vi "诊断标定3.vi"(8 "CAN端口":u16(ring), 9 "设备索引号":u16(ring), 10 "CAN卡类型":u32(ring)=21) -> ()   [LabVIEW 2013] (continued)
                                }
                                }
                                frame 8 {
                                n3916 = case shown="假" w5467 {
                                frame False {
                                n3917 = control-ref of="结果"() -> (w5470:refnum<vi>)
                                n3918 = Build Array("加热控制参数判定失败!") -> (w5471:string[])
                                n3919 = call "表格编辑.vi"("新元素/子数组"=w5471, "活动单元格:单元格背景色"=u32 16711680, "MCListbox引用句柄"=w5470) -> ()  [unwired: 9 out]
                                }
                                frame True {
                                }
                                }
                                }
                                frame 99, Default {
                                }
                                }
                                }
                              }
                            }
                          }
                        }
                        n3920 = disable-structure shown="禁用" {
                          frame Disabled {
                            n3921 = global read "读配置文件全局.vi" "SOC判定"() -> ()  [unwired: 1 out]
                          }
                          frame Enabled {
                          }
                        }
                      }
                    }
                  }
                  frame True {
                  }
                }
              }
            }
            n3922 = stacked-sequence {
              tunnel: w4698 -> [_]
              frame #0 {
                n3923 = local write "强制终止读写标记"(FALSE ("强制停止")) -> ()
              }
            }
            "重试次数" <- u8 0 ("重试次数")
          }
          frame "开启均衡" {
            n3924 = local read "从板板号"() -> (w5472:u8)
            n3925 = stacked-sequence {
              tunnel: 133 -> [_ w5498 _ _]
              tunnel: w5472 -> [_ _ _ _]
              frame #0 {
                w5482 = u8 0 items=["Normal", "Listen Only"] ("工作方式")
                w5481 = u8 1 items=["Dual Filter", "Single Filter"] ("滤波方式")
                n3926 = global write "EV05全局变量1.vi" "读取超时"(FALSE ("读取超时")) -> ()
                n3927 = global write "EV05全局变量1.vi" "流控帧 2"(TRUE ("流控帧 2")) -> ()
                n3928 = local write "写?"(TRUE ("写?")) -> ()
                n3929 = local read "设备索引号"() -> (w5477:u16)
                n3930 = local read "CAN卡类型"() -> (w5476:u32)
                n3931 = local read "CAN端口"() -> (w5478:u16)
                n3932 = local write "控制1"(TRUE ("控制1")) -> ()
                n3933 = local write "消除"(TRUE ("消除")) -> ()
                n3934 = global write "EV05全局变量1.vi" "流控帧"(FALSE ("流控帧")) -> ()
                n3935 = call "CAN_Init-8.6.vi"("CAN卡类型"=w5476, "设备索引号"=w5477, "CAN端口"=w5478, "操作类型"=enum16{"初始化CAN", "关闭CAN"}."初始化CAN", "滤波方式"=w5481, "Accept Code"=u32 606601216, "簇"=T21 {"打开CAN"=FALSE, "初始化CAN"=TRUE, "开始CAN"=TRUE, "重启"=FALSE, "关闭CAN"=FALSE}, "Mask Code"=u32 524287 ("Accept Code"), "工作方式"=w5482, "是否滤波"=TRUE, "滤波选择"=T20 {"fiter_mode"=1, "fiter_endid"=75825152, "fiter_startid"=75890687}) -> ()  [unwired: 3 in, 6 out]
                n3936 = Wait Until Next ms Multiple(millisecond multiple=u32 20 ("毫秒倍数")) -> ()  [unwired: 1 out]
              }
              frame #1 {
                n3937 = local write "命令"(w5498) -> ()
                n3938 = call "ID组合.vi"("SA(4)"=0 ("PDU(1)"), "PS(3)"=63 ("PDU(1)"), "PF(2)"=w5498, "PDU(1)"=4) -> ("ID"=w5497:i32)  [unwired: 7 out]
                n3939 = local read "均衡类型选择"() -> (w5494:enum16{"放电均衡", "充电均衡", "充放电均衡"})
                n3940 = local read "设备索引号"() -> (w5503:u16)
                n3941 = local read "CAN卡类型"() -> (w5504:u32)
                n3942 = local read "CAN端口"() -> (w5502:u16)
                n3943 = local write "命令序号"(2) -> ()
                n3944 = Add(x=w5494, y=1) -> (x+y=w5492:i32)
                n3945 = Build Array(2, 2, w5492) -> (w5505:i32[])
                n3946 = call "transmit-8.6.vi"("can卡类型"=w5504, "设备索引号"=w5503, "CAN端口"=w5502, "ID"=w5497, "SendType"=u8 0, "Data"=w5505) -> ()  [unwired: 3 in, 11 out]
              }
              frame #2 {
                n3947 = Wait Until Next ms Multiple(millisecond multiple=u32 1000 ("毫秒倍数")) -> ()  [unwired: 1 out]
              }
              frame #3 {
                w5513 = u8 0 items=["Normal", "Listen Only"] ("工作方式")
                w5514 = u8 1 items=["Dual Filter", "Single Filter"] ("滤波方式")
                n3948 = global write "EV05全局变量1.vi" "流控帧 2"(FALSE ("流控帧 2")) -> ()
                n3949 = local read "CAN卡类型"() -> (w5519:u32)
                n3950 = local read "设备索引号"() -> (w5518:u16)
                n3951 = local read "CAN端口"() -> (w5517:u16)
                n3952 = local write "控制1"(FALSE ("控制1")) -> ()
                n3953 = local write "消除"(FALSE ("消除")) -> ()
                n3954 = call <vilib>:"Unset Busy.vi"() -> ()  [unwired: 2 in, 10 out]
                n3955 = call "CAN_Init-8.6.vi"("CAN卡类型"=w5519, "设备索引号"=w5518, "CAN端口"=w5517, "操作类型"=enum16{"初始化CAN", "关闭CAN"}."初始化CAN", "滤波方式"=w5514, "Accept Code"=u32 3221225472, "簇"=T21 {"打开CAN"=FALSE, "初始化CAN"=TRUE, "开始CAN"=TRUE, "重启"=FALSE, "关闭CAN"=FALSE}, "Mask Code"=u32 1073741823 ("Accept Code"), "工作方式"=w5513, "是否滤波"=TRUE, "滤波选择"=T20 {"fiter_mode"=1, "fiter_endid"=402653184, "fiter_startid"=419430399}) -> ()  [unwired: 3 in, 6 out]
              }
            }
          }
          frame "关闭均衡" {
            n3956 = local read "从板板号"() -> (w5523:u8)
            n3957 = stacked-sequence {
              tunnel: 133 -> [_ w5547 _ _]
              tunnel: w5523 -> [_ _ _ _]
              frame #0 {
                w5533 = u8 0 items=["Normal", "Listen Only"] ("工作方式")
                w5532 = u8 1 items=["Dual Filter", "Single Filter"] ("滤波方式")
                n3958 = global write "EV05全局变量1.vi" "读取超时"(FALSE ("读取超时")) -> ()
                n3959 = global write "EV05全局变量1.vi" "流控帧 2"(TRUE ("流控帧 2")) -> ()
                n3960 = local write "写?"(TRUE ("写?")) -> ()
                n3961 = local read "设备索引号"() -> (w5528:u16)
                n3962 = local read "CAN卡类型"() -> (w5527:u32)
                n3963 = local read "CAN端口"() -> (w5529:u16)
                n3964 = local write "控制1"(TRUE ("控制1")) -> ()
                n3965 = global write "EV05全局变量1.vi" "流控帧"(FALSE ("流控帧")) -> ()
                n3966 = local write "消除"(TRUE ("消除")) -> ()
                n3967 = call "CAN_Init-8.6.vi"("CAN卡类型"=w5527, "设备索引号"=w5528, "CAN端口"=w5529, "操作类型"=enum16{"初始化CAN", "关闭CAN"}."初始化CAN", "滤波方式"=w5532, "Accept Code"=u32 606601216, "簇"=T21 {"打开CAN"=FALSE, "初始化CAN"=TRUE, "开始CAN"=TRUE, "重启"=FALSE, "关闭CAN"=FALSE}, "Mask Code"=u32 524287 ("Accept Code"), "工作方式"=w5533, "是否滤波"=TRUE, "滤波选择"=T20 {"fiter_mode"=1, "fiter_endid"=75825152, "fiter_startid"=75890687}) -> ()  [unwired: 3 in, 6 out]
                n3968 = Wait Until Next ms Multiple(millisecond multiple=u32 20 ("毫秒倍数")) -> ()  [unwired: 1 out]
              }
              frame #1 {
                n3969 = local write "命令"(w5547) -> ()
                n3970 = call "ID组合.vi"("SA(4)"=0 ("PDU(1)"), "PS(3)"=63 ("PDU(1)"), "PF(2)"=w5547, "PDU(1)"=4) -> ("ID"=w5546:i32)  [unwired: 7 out]
                n3971 = local read "均衡类型选择"() -> (w5557:enum16{"放电均衡", "充电均衡", "充放电均衡"})
                n3972 = local write "命令序号"(3) -> ()
                n3973 = local read "设备索引号"() -> (w5552:u16)
                n3974 = local read "CAN卡类型"() -> (w5553:u32)
                n3975 = local read "CAN端口"() -> (w5551:u16)
                n3976 = Add(x=w5557, y=1) -> (x+y=w5555:i32)
                n3977 = Build Array(2, 3, w5555) -> (w5554:i32[])
                n3978 = call "transmit-8.6.vi"("can卡类型"=w5553, "设备索引号"=w5552, "CAN端口"=w5551, "ID"=w5546, "SendType"=u8 0, "Data"=w5554) -> ()  [unwired: 3 in, 11 out]
              }
              frame #2 {
                n3979 = Wait Until Next ms Multiple(millisecond multiple=u32 1000 ("毫秒倍数")) -> ()  [unwired: 1 out]
              }
              frame #3 {
                w5564 = u8 0 items=["Normal", "Listen Only"] ("工作方式")
                w5565 = u8 1 items=["Dual Filter", "Single Filter"] ("滤波方式")
                n3980 = local read "设备索引号"() -> (w5569:u16)
                n3981 = local read "CAN卡类型"() -> (w5570:u32)
                n3982 = global write "EV05全局变量1.vi" "流控帧 2"(FALSE ("流控帧 2")) -> ()
                n3983 = local read "CAN端口"() -> (w5568:u16)
                n3984 = local write "控制1"(FALSE ("控制1")) -> ()
                n3985 = local write "消除"(FALSE ("消除")) -> ()
                n3986 = call "CAN_Init-8.6.vi"("CAN卡类型"=w5570, "设备索引号"=w5569, "CAN端口"=w5568, "操作类型"=enum16{"初始化CAN", "关闭CAN"}."初始化CAN", "滤波方式"=w5565, "Accept Code"=u32 3221225472, "簇"=T21 {"打开CAN"=FALSE, "初始化CAN"=TRUE, "开始CAN"=TRUE, "重启"=FALSE, "关闭CAN"=FALSE}, "Mask Code"=u32 1073741823 ("Accept Code"), "工作方式"=w5564, "是否滤波"=TRUE, "滤波选择"=T20 {"fiter_mode"=1, "fiter_endid"=402653184, "fiter_startid"=419430399}) -> ()  [unwired: 3 in, 6 out]
                n3987 = call <vilib>:"Unset Busy.vi"() -> ()  [unwired: 2 in, 10 out]
              }
            }
          }
          frame "强制均衡" {
            n3988 = local read "从板板号"() -> (w5574:u8)
            n3989 = stacked-sequence {
              tunnel: 133 -> [_ w5605 _ _]
              tunnel: w5574 -> [_ _ _ _]
              frame #0 {
                w5584 = u8 0 items=["Normal", "Listen Only"] ("工作方式")
                w5583 = u8 1 items=["Dual Filter", "Single Filter"] ("滤波方式")
                n3990 = global write "EV05全局变量1.vi" "读取超时"(FALSE ("读取超时")) -> ()
                n3991 = global write "EV05全局变量1.vi" "流控帧 2"(TRUE ("流控帧 2")) -> ()
                n3992 = local write "写?"(TRUE ("写?")) -> ()
                n3993 = local read "设备索引号"() -> (w5579:u16)
                n3994 = local read "CAN卡类型"() -> (w5578:u32)
                n3995 = local write "控制1"(TRUE ("控制1")) -> ()
                n3996 = local read "CAN端口"() -> (w5580:u16)
                n3997 = local write "消除"(TRUE ("消除")) -> ()
                n3998 = global write "EV05全局变量1.vi" "流控帧"(FALSE ("流控帧")) -> ()
                n3999 = call "CAN_Init-8.6.vi"("CAN卡类型"=w5578, "设备索引号"=w5579, "CAN端口"=w5580, "操作类型"=enum16{"初始化CAN", "关闭CAN"}."初始化CAN", "滤波方式"=w5583, "Accept Code"=u32 606601216, "簇"=T21 {"打开CAN"=FALSE, "初始化CAN"=TRUE, "开始CAN"=TRUE, "重启"=FALSE, "关闭CAN"=FALSE}, "Mask Code"=u32 524287 ("Accept Code"), "工作方式"=w5584, "是否滤波"=TRUE, "滤波选择"=T20 {"fiter_mode"=1, "fiter_endid"=75825152, "fiter_startid"=75890687}) -> ()  [unwired: 3 in, 6 out]
                n4000 = Wait Until Next ms Multiple(millisecond multiple=u32 20 ("毫秒倍数")) -> ()  [unwired: 1 out]
              }
              frame #1 {
                n4001 = local read "强制类型"() -> (w5611:enum16{"全通道开启", "单通道开启", "清待均衡时间"})
                n4002 = case shown="\"清待均衡时间\"" w5611 {
                  tunnel: [250 252 254] -> w5601
                  tunnel: [_ w5630 _] -> w5600
                  tunnel: [_ w5629 _] -> w5599
                  tunnel: [_ w5620 _] -> w5598
                  tunnel: [_ w5613 _] -> w5597
                  frame "全通道开启", Default {
                  }
                  frame "单通道开启" {
                    n4003 = local read "均衡类型选择"() -> (w5628:enum16{"放电均衡", "充电均衡", "充放电均衡"})
                    n4004 = local read "均衡位置"() -> (w5623:u16)
                    n4005 = case shown="\"放电均衡\", 默认" w5628 {
                      tunnel: [0 1] -> w5627
                      frame "放电均衡", Default {
                      }
                      frame "充电均衡" {
                      }
                    }
                    n4006 = Multiply(x="均衡时间", y=6.0) -> (x*y=w5615:dbl)
                    n4007 = Quotient & Remainder(x=w5615, y=256.0) -> (x-y*floor(x/y)=w5613:dbl, floor(x/y)=w5614:dbl)
                    n4008 = call "二进制解析-8.6.vi"("索引"=1, "数值"=w5627) -> ("低位子数组"=w5618:i32[])  [unwired: 1 in, 2 out]
                    n4009 = Quotient & Remainder(x=w5623, y=256.0) -> (x-y*floor(x/y)=w5629:dbl, floor(x/y)=w5630:dbl)
                    n4010 = call "二进制解析-8.6.vi"("索引"=8, "数值"=w5614) -> ("低位子数组"=w5619:i32[])  [unwired: 1 in, 2 out]
                    n4011 = Replace Array Subset(array=w5619, new element=w5618, index=0 ("索引")) -> (w5616:i32[])
                    n4012 = call "数值二进制转十进制-8.6.vi"("子数组"=w5616) -> ("十进制数值"=w5620:i32)  [unwired: 4 in]
                  }
                  frame "清待均衡时间" {
                  }
                }
                n4013 = local write "命令"(w5605) -> ()
                n4014 = call "ID组合.vi"("SA(4)"=0 ("PDU(1)"), "PS(3)"=63 ("PDU(1)"), "PF(2)"=w5605, "PDU(1)"=4) -> ("ID"=w5604:i32)  [unwired: 7 out]
                n4015 = local read "设备索引号"() -> (w5608:u16)
                n4016 = local read "CAN卡类型"() -> (w5609:u32)
                n4017 = local read "CAN端口"() -> (w5607:u16)
                n4018 = local write "命令序号"(w5601) -> ()
                n4019 = Build Array(6, 4, w5601, w5600, w5599, w5598, w5597) -> (w5610:dbl[])
                n4020 = call "transmit-8.6.vi"("can卡类型"=w5609, "设备索引号"=w5608, "CAN端口"=w5607, "ID"=w5604, "SendType"=u8 0, "Data"=w5610) -> ()  [unwired: 3 in, 11 out]
              }
              frame #2 {
                n4021 = Wait Until Next ms Multiple(millisecond multiple=u32 1000 ("毫秒倍数")) -> ()  [unwired: 1 out]
              }
              frame #3 {
                w5644 = u8 0 items=["Normal", "Listen Only"] ("工作方式")
                w5643 = u8 1 items=["Dual Filter", "Single Filter"] ("滤波方式")
                n4022 = global write "EV05全局变量1.vi" "流控帧 2"(FALSE ("流控帧 2")) -> ()
                n4023 = local write "控制1"(FALSE ("控制1")) -> ()
                n4024 = local read "设备索引号"() -> (w5639:u16)
                n4025 = local read "CAN卡类型"() -> (w5638:u32)
                n4026 = local write "消除"(FALSE ("消除")) -> ()
                n4027 = local read "CAN端口"() -> (w5640:u16)
                n4028 = call <vilib>:"Unset Busy.vi"() -> ()  [unwired: 2 in, 10 out]
                n4029 = call "CAN_Init-8.6.vi"("CAN卡类型"=w5638, "设备索引号"=w5639, "CAN端口"=w5640, "操作类型"=enum16{"初始化CAN", "关闭CAN"}."初始化CAN", "滤波方式"=w5643, "Accept Code"=u32 3221225472, "簇"=T21 {"打开CAN"=FALSE, "初始化CAN"=TRUE, "开始CAN"=TRUE, "重启"=FALSE, "关闭CAN"=FALSE}, "Mask Code"=u32 1073741823 ("Accept Code"), "工作方式"=w5644, "是否滤波"=TRUE, "滤波选择"=T20 {"fiter_mode"=1, "fiter_endid"=402653184, "fiter_startid"=419430399}) -> ()  [unwired: 3 in, 6 out]
              }
            }
          }
          frame "项目软件版本读取" {
            n4030 = stacked-sequence {
              seq-local: [_ w5665 _] -> [_ _ w5672]
              frame #0 {
                n4031 = local read "设备索引号"() -> (w5652:u16)
                n4032 = local read "CAN卡类型"() -> (w5653:u32)
                n4033 = local read "CAN端口"() -> (w5651:u16)
                n4034 = stacked-sequence {
                  tunnel: w5653 -> [w5656 w5664]
                  tunnel: w5652 -> [w5655 w5663]
                  tunnel: w5651 -> [w5654 w5662]
                  frame #0 {
                    n4035 = dll-call lib="PTH1tabs FBluewave New EnergySVN_Work\nBNET01_BMStrunkBMS_Monitor_增加二维码data\nkerneldlls\nusbcan.dll" fn="VCI_ClearBuffer"("DeviceType"=w5656, "DeviceInd"=w5655, "CANInd"=w5654) -> (error out=w5657:errorcluster)  [unwired: 4 in, 4 out]
                    n4036 = call <vilib>:"Clear Errors.vi"("error in (no error)"=w5657) -> ()  [unwired: 6 in, 1 out]
                  }
                  frame #1 {
                    w5661 = u8 137 ("命令")
                    w5660 = u32 1 ("命令序号")
                    n4037 = local read "从板板号"() -> (w5658:u8)
                    n4038 = local write "命令"(w5661) -> ()
                    n4039 = call "多帧发送机制(EV05).vi"("can卡类型"=w5664, "设备索引号"=w5663, "CAN端口"=w5662, "命令"=w5661, "板号"=w5658, "命令序号"=w5660, "输入数据"=dbl[] [0.0]) -> ()  [unwired: 1 in, 12 out]
                    n4040 = local write "命令序号"(w5660) -> ()
                  }
                }
              }
              frame #1 {
                n4041 = while {
                  tunnel: [w5666] -> w5665
                  i -> [w5671]
                  stop <- w5668 stop-if-true
                  n4042 = global read "EV05全局变量1.vi" "写入超时"() -> (w5666:bool)
                  n4043 = Greater Or Equal?(x=w5671, y=25) -> (x >= y?=w5669:bool)
                  n4044 = Or(x=w5666, y=w5669) -> (x .or. y?=w5668:bool)
                  n4045 = Wait Until Next ms Multiple(millisecond multiple=u32 100 ("毫秒倍数")) -> ()  [unwired: 1 out]
                }
              }
              frame #2 {
                n4046 = case shown="假" w5672 {
                  frame False {
                    n4047 = control-ref of="结果"() -> (w5674:refnum<vi>)
                    n4048 = Concatenate Strings("项目软件版本" ("字符串"), "     读取失败" ("字符串")) -> (w5677:string)
                    n4049 = Build Array(w5677) -> (w5676:string[])
                    n4050 = call "表格编辑(版本读取).vi"("新元素/子数组"=w5676, "活动单元格:单元格背景色"=u32 16740749, "MCListbox引用句柄"=w5674) -> ()  [unwired: 9 out]
                  }
                  frame True {
                  }
                }
                n4051 = call <vilib>:"Unset Busy.vi"() -> ()  [unwired: 2 in, 10 out]
              }
            }
          }
          frame "读取故障状态" {
            n4052 = stacked-sequence {
              seq-local: [_ w5703 _] -> [_ _ w5710]
              frame #0 {
                n4053 = local read "设备索引号"() -> (w5680:u16)
                n4054 = local read "CAN卡类型"() -> (w5681:u32)
                n4055 = local read "CAN端口"() -> (w5679:u16)
                n4056 = stacked-sequence {
                  tunnel: w5681 -> [w5684 w5693]
                  tunnel: w5680 -> [w5683 w5692]
                  tunnel: w5679 -> [w5682 w5691]
                  frame #0 {
                    n4057 = dll-call lib="PTH1tabs FBluewave New EnergySVN_Work\nBNET01_BMStrunkBMS_Monitor_增加二维码data\nkerneldlls\nusbcan.dll" fn="VCI_ClearBuffer"("DeviceType"=w5684, "DeviceInd"=w5683, "CANInd"=w5682) -> (error out=w5685:errorcluster)  [unwired: 4 in, 4 out]
                    n4058 = call <vilib>:"Clear Errors.vi"("error in (no error)"=w5685) -> ()  [unwired: 6 in, 1 out]
                  }
                  frame #1 {
                    n4059 = local read "从板板号 2"() -> (w5686:u8)
                    n4060 = case shown="1..30" w5686 {
                      tunnel: [u8 133 ("命令") u8 4 ("命令")] -> w5690
                      frame 0, Default {
                      }
                      frame 1..30 {
                      }
                    }
                    n4061 = local read "状态选择"() -> (w5688:T18)
                    n4062 = local write "命令"(w5690) -> ()
                    n4063 = case shown="\"预充电故障,继电器驱动故障\"" w5688 {
                      tunnel: [1 2 3 4 5 6 7] -> w5687
                      frame "电压,内总电压,外总电压,温度,电流,绝缘,系统时钟,充电均衡,放电均衡", Default {
                      }
                      frame "CPU,CPU内部EE存储器,CPU内部FLASH,内部EE存储器,45db存储器" {
                      }
                      frame "CAN检测故障" {
                      }
                      frame "软件故障" {
                      }
                      frame "RS485,RS232检测故障" {
                      }
                      frame "DI,DO,AI,AO检测故障" {
                      }
                      frame "预充电故障,继电器驱动故障" {
                      }
                    }
                    n4064 = call "多帧发送机制(EV05).vi"("can卡类型"=w5693, "设备索引号"=w5692, "CAN端口"=w5691, "命令"=w5690, "板号"=w5686, "命令序号"=w5687, "输入数据"=dbl[] [0.0]) -> ()  [unwired: 1 in, 12 out]
                    n4065 = local write "命令序号"(w5687) -> ()
                  }
                }
              }
              frame #1 {
                n4066 = while {
                  tunnel: [w5704] -> w5703
                  i -> [w5709]
                  stop <- w5706 stop-if-true
                  n4067 = global read "EV05全局变量1.vi" "写入超时"() -> (w5704:bool)
                  n4068 = Greater Or Equal?(x=w5709, y=25) -> (x >= y?=w5707:bool)
                  n4069 = Or(x=w5704, y=w5707) -> (x .or. y?=w5706:bool)
                  n4070 = Wait Until Next ms Multiple(millisecond multiple=u32 100 ("毫秒倍数")) -> ()  [unwired: 1 out]
                }
              }
              frame #2 {
                n4071 = case shown="真" w5710 {
                  frame False {
                    n4072 = Concatenate Strings("故障信息" ("字符串"), "     读取失败" ("字符串")) -> (w5712:string)
                    n4073 = One Button Dialog(message=w5712, button name ("OK")="确定" ("按钮名称（“确定”）")) -> ()  [unwired: 1 out]
                  }
                  frame True {
                    n4074 = One Button Dialog(message="故障信息读取完成" ("字符串"), button name ("OK")="确定" ("按钮名称（“确定”）")) -> ()  [unwired: 1 out]
                  }
                }
                n4075 = call <vilib>:"Unset Busy.vi"() -> ()  [unwired: 2 in, 10 out]
              }
            }
          }
          frame "平台软件版本读取" {
            n4076 = stacked-sequence {
              seq-local: [_ w5732 _] -> [_ _ w5739]
              frame #0 {
                n4077 = local read "设备索引号"() -> (w5719:u16)
                n4078 = local read "CAN卡类型"() -> (w5720:u32)
                n4079 = local read "CAN端口"() -> (w5718:u16)
                n4080 = stacked-sequence {
                  tunnel: w5720 -> [w5723 w5731]
                  tunnel: w5719 -> [w5722 w5730]
                  tunnel: w5718 -> [w5721 w5729]
                  tunnel: u8 137 ("命令") -> [_ w5728]
                  frame #0 {
                    n4081 = dll-call lib="PTH1tabs FBluewave New EnergySVN_Work\nBNET01_BMStrunkBMS_Monitor_增加二维码data\nkerneldlls\nusbcan.dll" fn="VCI_ClearBuffer"("DeviceType"=w5723, "DeviceInd"=w5722, "CANInd"=w5721) -> (error out=w5724:errorcluster)  [unwired: 4 in, 4 out]
                    n4082 = call <vilib>:"Clear Errors.vi"("error in (no error)"=w5724) -> ()  [unwired: 6 in, 1 out]
                  }
                  frame #1 {
                    w5727 = u32 2 ("命令序号")
                    n4083 = local read "从板板号"() -> (w5725:u8)
                    n4084 = local write "命令"(w5728) -> ()
                    n4085 = call "多帧发送机制(EV05).vi"("can卡类型"=w5731, "设备索引号"=w5730, "CAN端口"=w5729, "命令"=w5728, "板号"=w5725, "命令序号"=w5727, "输入数据"=dbl[] [0.0]) -> ()  [unwired: 1 in, 12 out]
                    n4086 = local write "命令序号"(w5727) -> ()
                  }
                }
              }
              frame #1 {
                n4087 = while {
                  tunnel: [w5733] -> w5732
                  i -> [w5738]
                  stop <- w5735 stop-if-true
                  n4088 = global read "EV05全局变量1.vi" "写入超时"() -> (w5733:bool)
                  n4089 = Greater Or Equal?(x=w5738, y=25) -> (x >= y?=w5736:bool)
                  n4090 = Or(x=w5733, y=w5736) -> (x .or. y?=w5735:bool)
                  n4091 = Wait Until Next ms Multiple(millisecond multiple=u32 100 ("毫秒倍数")) -> ()  [unwired: 1 out]
                }
              }
              frame #2 {
                n4092 = case shown="假" w5739 {
                  frame False {
                    n4093 = control-ref of="结果"() -> (w5742:refnum<vi>)
                    n4094 = Concatenate Strings("平台软件版本" ("字符串"), "     读取失败" ("字符串")) -> (w5744:string)
                    n4095 = Build Array(w5744) -> (w5741:string[])
                    n4096 = call "表格编辑(版本读取).vi"("新元素/子数组"=w5741, "活动单元格:单元格背景色"=u32 16740749, "MCListbox引用句柄"=w5742) -> ()  [unwired: 9 out]
                  }
                  frame True {
                  }
                }
                n4097 = call <vilib>:"Unset Busy.vi"() -> ()  [unwired: 2 in, 10 out]
              }
            }
          }
          frame "模块软件版本读取" {
            n4098 = local read "从板板号"() -> (w5746:u8)
            n4099 = local read "模块软件版本"() -> (w5747:T1)
            n4100 = case shown="\"全部读取\"" w5747 {
              selector: w5747 -> [w5748 w5792]
              tunnel: w5746 -> [_ w5791]
              frame "BCUMCAL", Default {
                n4101 = stacked-sequence {
                  seq-local: [_ _ w5774 _] -> [_ _ _ w5781]
                  tunnel: w5748 -> [_ w5754 _ w5782]
                  frame #0 {
                    w5753 = FALSE ("写?")
                    n4102 = call <vilib>:"Set Busy.vi"("disable click? (T)"=FALSE) -> ()  [unwired: 3 in, 8 out]
                    n4103 = local write "写?"(w5753) -> ()
                    n4104 = global write "EV05全局变量1.vi" "流控帧 2"(TRUE ("流控帧 2")) -> ()
                    n4105 = global write "EV05全局变量1.vi" "写入超时"(w5753) -> ()
                    n4106 = local write "控制1"(TRUE ("控制1")) -> ()
                    n4107 = local write "消除"(TRUE ("消除")) -> ()
                  }
                  frame #1 {
                    n4108 = Quotient & Remainder(x=w5754, y=256) -> (x-y*floor(x/y)=w5755:i32, floor(x/y)=w5756:i32)
                    n4109 = Build Array(w5756, w5755, u8 0 ("板号")) -> (w5759:i32[])
                    n4110 = local read "设备索引号"() -> (w5761:u16)
                    n4111 = local read "CAN卡类型"() -> (w5762:u32)
                    n4112 = local read "CAN端口"() -> (w5760:u16)
                    n4113 = stacked-sequence {
                      tunnel: w5762 -> [w5765 w5773]
                      tunnel: w5761 -> [w5764 w5772]
                      tunnel: w5760 -> [w5763 w5771]
                      tunnel: w5759 -> [_ w5770]
                      frame #0 {
                        n4114 = dll-call lib="PTH1tabs FBluewave New EnergySVN_Work\nBNET01_BMStrunkBMS_Monitor_增加二维码data\nkerneldlls\nusbcan.dll" fn="VCI_ClearBuffer"("DeviceType"=w5765, "DeviceInd"=w5764, "CANInd"=w5763) -> (error out=w5766:errorcluster)  [unwired: 4 in, 4 out]
                        n4115 = call <vilib>:"Clear Errors.vi"("error in (no error)"=w5766) -> ()  [unwired: 6 in, 1 out]
                      }
                      frame #1 {
                        w5769 = u8 137 ("命令")
                        w5767 = u32 3 ("命令序号")
                        n4116 = local read "从板板号"() -> (w5768:u8)
                        n4117 = local write "命令"(w5769) -> ()
                        n4118 = call "多帧发送机制(EV05).vi"("can卡类型"=w5773, "设备索引号"=w5772, "CAN端口"=w5771, "命令"=w5769, "板号"=w5768, "命令序号"=w5767, "输入数据"=w5770) -> ()  [unwired: 1 in, 12 out]
                        n4119 = local write "命令序号"(w5767) -> ()
                      }
                    }
                  }
                  frame #2 {
                    n4120 = while {
                      tunnel: [w5775] -> w5774
                      i -> [w5780]
                      stop <- w5776 stop-if-true
                      n4121 = global read "EV05全局变量1.vi" "写入超时"() -> (w5775:bool)
                      n4122 = Greater Or Equal?(x=w5780, y=25) -> (x >= y?=w5777:bool)
                      n4123 = Or(x=w5775, y=w5777) -> (x .or. y?=w5776:bool)
                      n4124 = Wait Until Next ms Multiple(millisecond multiple=u32 100 ("毫秒倍数")) -> ()  [unwired: 1 out]
                    }
                  }
                  frame #3 {
                    n4125 = call <vilib>:"Unset Busy.vi"() -> ()  [unwired: 2 in, 10 out]
                    n4126 = case shown="假" w5781 {
                      tunnel: w5782 -> [w5784 _]
                      frame False {
                        n4127 = Number To Decimal String(number=w5784) -> (decimal integer string=w5785:string)  [unwired: 1 out]
                        n4128 = control-ref of="结果"() -> (w5786:refnum<vi>)
                        n4129 = Concatenate Strings("模块" ("字符串"), w5785, "     读取失败" ("字符串")) -> (w5789:string)
                        n4130 = Build Array(w5789) -> (w5788:string[])
                        n4131 = call "表格编辑(版本读取).vi"("新元素/子数组"=w5788, "活动单元格:单元格背景色"=u32 16740749, "MCListbox引用句柄"=w5786) -> ()  [unwired: 9 out]
                      }
                      frame True {
                      }
                    }
                  }
                }
              }
              frame "全部读取" {
                n4132 = stacked-sequence {
                  seq-local: [w5793 _] -> [_ w5831]
                  tunnel: w5792 -> [_ w5833]
                  tunnel: w5791 -> [w5794 w5832]
                  frame #0 {
                    n4133 = stacked-sequence {
                      tunnel: w5794 -> [_ w5803 _]
                      tunnel: [_ _ w5823] -> w5793
                      frame #0 {
                        w5799 = FALSE ("写?")
                        n4134 = control-ref of="模块软件版本 2"() -> (w5797:refnum<vi>)
                        n4135 = call <vilib>:"Set Busy.vi"("disable click? (T)"=FALSE) -> ()  [unwired: 3 in, 8 out]
                        n4136 = local write "写?"(w5799) -> ()
                        n4137 = property class="MCListbox (严格)"(reference=w5797, "ItemNames"=string[][] []) -> ()  [unwired: 1 in, 2 out]
                        n4138 = global write "EV05全局变量1.vi" "写入超时"(w5799) -> ()
                        n4139 = local write "消除"(TRUE ("消除")) -> ()
                        n4140 = global write "EV05全局变量1.vi" "流控帧 2"(TRUE ("流控帧 2")) -> ()
                        n4141 = local write "控制1"(TRUE ("控制1")) -> ()
                        n4142 = local write "MODEL号"(u8[] [] ("MODEL号")) -> ()
                      }
                      frame #1 {
                        n4143 = local read "设备索引号"() -> (w5805:u16)
                        n4144 = local read "CAN卡类型"() -> (w5806:u32)
                        n4145 = local read "CAN端口"() -> (w5804:u16)
                        n4146 = stacked-sequence {
                          tunnel: w5806 -> [w5809 w5822]
                          tunnel: w5805 -> [w5808 w5821]
                          tunnel: w5804 -> [w5807 w5820]
                          tunnel: w5803 -> [_ w5812]
                          frame #0 {
                            n4147 = dll-call lib="PTH1tabs FBluewave New EnergySVN_Work\nBNET01_BMStrunkBMS_Monitor_增加二维码data\nkerneldlls\nusbcan.dll" fn="VCI_ClearBuffer"("DeviceType"=w5809, "DeviceInd"=w5808, "CANInd"=w5807) -> (error out=w5810:errorcluster)  [unwired: 4 in, 4 out]
                            n4148 = call <vilib>:"Clear Errors.vi"("error in (no error)"=w5810) -> ()  [unwired: 6 in, 1 out]
                          }
                          frame #1 {
                            w5818 = u8 137 ("命令")
                            w5816 = u32 3 ("命令序号")
                            n4149 = Quotient & Remainder(x=u8 0 ("板号"), y=256) -> (x-y*floor(x/y)=w5813:i32, floor(x/y)=w5814:i32)
                            n4150 = local write "命令"(w5818) -> ()
                            n4151 = Build Array(w5814, w5813, u8 0 ("板号")) -> (w5819:i32[])
                            n4152 = call "多帧发送机制(EV05).vi"("can卡类型"=w5822, "设备索引号"=w5821, "CAN端口"=w5820, "命令"=w5818, "板号"=w5812, "命令序号"=w5816, "输入数据"=w5819) -> ()  [unwired: 1 in, 12 out]
                            n4153 = local write "命令序号"(w5816) -> ()
                          }
                        }
                      }
                      frame #2 {
                        n4154 = while {
                          tunnel: [w5825] -> w5823
                          i -> [w5829]
                          stop <- w5826 stop-if-true
                          n4155 = local read "强制停止版本读取"() -> (w5824:bool)
                          n4156 = global read "EV05全局变量1.vi" "写入超时"() -> (w5825:bool)
                          n4157 = Greater Or Equal?(x=w5829, y=35) -> (x >= y?=w5827:bool)
                          n4158 = Compound Arithmetic op=OR(w5824, w5825, w5827) -> (w5826:bool)
                          n4159 = Wait Until Next ms Multiple(millisecond multiple=u32 100 ("毫秒倍数")) -> ()  [unwired: 1 out]
                        }
                      }
                    }
                  }
                  frame #1 {
                    n4160 = case shown="真" w5831 {
                      tunnel: w5833 -> [_ w5843]
                      tunnel: w5832 -> [_ w5842]
                      frame False {
                        n4161 = control-ref of="结果"() -> (w5835:refnum<vi>)
                        n4162 = Concatenate Strings("模块编号" ("字符串"), "读取失败" ("字符串")) -> (w5838:string)
                        n4163 = Build Array(w5838) -> (w5837:string[])
                        n4164 = call "表格编辑(版本读取).vi"("新元素/子数组"=w5837, "活动单元格:单元格背景色"=u32 16740749, "MCListbox引用句柄"=w5835) -> ()  [unwired: 9 out]
                        n4165 = call <vilib>:"Unset Busy.vi"() -> ()  [unwired: 11 in, 1 out]
                      }
                      frame True {
                        n4166 = local read "MODEL号"() -> (w5841:u8[])
                        n4167 = Array Size(array=w5841) -> (size(s)=w5840:i32)
                        n4168 = for {
                          tunnel: w5843 -> [_]
                          tunnel: w5842 -> [w5846]
                          tunnel: w5841 -> [w5845] mode=indexing
                          tunnel: w5840 -> [w5844]
                          i -> [w5848]
                          n4169 = Increment(x=w5848) -> (x+1=w5847:i32)
                          n4170 = stacked-sequence {
                            seq-local: [_ _ _ w5875 _ _] -> [_ _ _ _ w5884 _]
                            seq-local: [_ w5854 _ _ _ _] -> [_ _ _ _ w5883 _]
                            tunnel: w5847 -> [_ _ _ _ _ w5895]
                            tunnel: w5845 -> [_ w5854 _ _ _ _]
                            tunnel: w5846 -> [_ w5855 _ _ _ _]
                            tunnel: w5844 -> [_ _ _ _ _ w5893]
                            frame #0 {
                              w5850 = FALSE ("写?")
                              n4171 = call <vilib>:"Set Busy.vi"("disable click? (T)"=FALSE) -> ()  [unwired: 3 in, 8 out]
                              n4172 = local write "写?"(w5850) -> ()
                              n4173 = global write "EV05全局变量1.vi" "写入超时"(w5850) -> ()
                              n4174 = global write "EV05全局变量1.vi" "流控帧 2"(TRUE ("流控帧 2")) -> ()
                              n4175 = local write "控制1"(TRUE ("控制1")) -> ()
                              n4176 = local write "消除"(TRUE ("消除")) -> ()
                            }
                            frame #1 {
                              n4177 = local read "设备索引号"() -> (w5857:u16)
                              n4178 = local read "CAN卡类型"() -> (w5858:u32)
                              n4179 = local read "CAN端口"() -> (w5856:u16)
                              n4180 = stacked-sequence {
                                tunnel: w5858 -> [w5861 w5874]
                                tunnel: w5857 -> [w5860 w5873]
                                tunnel: w5856 -> [w5859 w5872]
                                tunnel: w5855 -> [_ w5864]
                                tunnel: w5854 -> [_ w5863]
                                frame #0 {
                                n4181 = dll-call lib="PTH1tabs FBluewave New EnergySVN_Work\nBNET01_BMStrunkBMS_Monitor_增加二维码data\nkerneldlls\nusbcan.dll" fn="VCI_ClearBuffer"("DeviceType"=w5861, "DeviceInd"=w5860, "CANInd"=w5859) -> (error out=w5862:errorcluster)  [unwired: 4 in, 4 out]
                                n4182 = call <vilib>:"Clear Errors.vi"("error in (no error)"=w5862) -> ()  [unwired: 6 in, 1 out]
                                }
                                frame #1 {
                                w5870 = u8 137 ("命令")
                                w5868 = u32 3 ("命令序号")
                                n4183 = Quotient & Remainder(x=w5863, y=256) -> (x-y*floor(x/y)=w5865:i32, floor(x/y)=w5866:i32)
                                n4184 = local write "命令"(w5870) -> ()
                                n4185 = Build Array(w5866, w5865, u8 0 ("板号")) -> (w5871:i32[])
                                n4186 = call "多帧发送机制(EV05).vi"("can卡类型"=w5874, "设备索引号"=w5873, "CAN端口"=w5872, "命令"=w5870, "板号"=w5864, "命令序号"=w5868, "输入数据"=w5871) -> ()  [unwired: 1 in, 12 out]
                                n4187 = local write "命令序号"(w5868) -> ()
                                }
                              }
                            }
                            frame #2 {
                            }
                            frame #3 {
                              n4188 = while {
                                tunnel: [w5877] -> w5875
                                i -> [w5881]
                                stop <- w5878 stop-if-true
                                n4189 = local read "强制停止版本读取"() -> (w5876:bool)
                                n4190 = global read "EV05全局变量1.vi" "写入超时"() -> (w5877:bool)
                                n4191 = Greater Or Equal?(x=w5881, y=25) -> (x >= y?=w5879:bool)
                                n4192 = Compound Arithmetic op=OR(w5876, w5877, w5879) -> (w5878:bool)
                                n4193 = Wait Until Next ms Multiple(millisecond multiple=u32 100 ("毫秒倍数")) -> ()  [unwired: 1 out]
                              }
                            }
                            frame #4 {
                              n4194 = call <vilib>:"Unset Busy.vi"() -> ()  [unwired: 11 in, 1 out]
                              n4195 = case shown="假" w5884 {
                                tunnel: w5883 -> [w5886 _]
                                frame False {
                                n4196 = control-ref of="结果"() -> (w5888:refnum<vi>)
                                n4197 = Number To Decimal String(number=w5886) -> (decimal integer string=w5887:string)  [unwired: 1 out]
                                n4198 = Concatenate Strings("模块" ("字符串"), w5887, "     读取失败" ("字符串")) -> (w5891:string)
                                n4199 = Build Array(w5891) -> (w5890:string[])
                                n4200 = call "表格编辑(版本读取).vi"("新元素/子数组"=w5890, "活动单元格:单元格背景色"=u32 16740749, "MCListbox引用句柄"=w5888) -> ()  [unwired: 9 out]
                                }
                                frame True {
                                }
                              }
                            }
                            frame #5 {
                              n4201 = Equal?(x=w5893, y=w5895) -> (x = y?=w5894:bool)
                              n4202 = case shown="真" w5894 {
                                frame False {
                                }
                                frame True {
                                n4203 = control-ref of="模块软件版本 2"() -> (w5906:refnum<vi>)
                                n4204 = local read "模块版本名称"() -> (w5905:string[][])
                                n4205 = local read "模块版本值"() -> (w5901:string[][])
                                n4206 = control-ref of="结果"() -> (w5913:refnum<vi>)
                                n4207 = property class="MCListbox (严格)"(reference=w5906) -> ("ItemNames"=w5909:string[][])  [unwired: 1 in, 2 out]
                                n4208 = local read "从板板号"() -> (w5896:u8)
                                n4209 = Concatenate Strings("模块版本读取完成" ("字符串")) -> (w5916:string)
                                n4210 = Build Array(w5916) -> (w5915:string[])
                                n4211 = call "表格编辑(版本读取).vi"("新元素/子数组"=w5915, "活动单元格:单元格背景色"=u32 21937, "MCListbox引用句柄"=w5913) -> ()  [unwired: 9 out]
                                n4212 = Transpose 2D Array(2D array=w5909) -> (transposed array=w5910:string[][])
                                n4213 = local write "强制停止版本读取"(FALSE ("强制停止 2")) -> ()
                                n4214 = local read "模块个数"() -> (w5899:u8[])
                                n4215 = Index Array(array=w5910, index (row) #1=0 ("索引 (行)"), index (row) #2=1 ("索引 (行)")) -> (element #1=w5900:string[], element #2=w5902:string[])  [unwired: 2 in]
                                n4216 = Replace Array Subset(array=w5905, new element=w5900, index (row)=w5896) -> (w5904:string[][])  [unwired: 1 in]
                                n4217 = Replace Array Subset(array=w5901, new element=w5902, index (row)=w5896) -> (w5903:string[][])  [unwired: 1 in]
                                n4218 = local write "模块版本名称"(w5904) -> ()
                                n4219 = local write "模块版本值"(w5903) -> ()
                                n4220 = Array Size(array=w5900) -> (size(s)=w5897:i32)
                                n4221 = Replace Array Subset(array=w5899, new element=w5897, index=w5896) -> (w5898:u8[])
                                n4222 = local write "模块个数"(w5898) -> ()
                                }
                              }
                            }
                          }
                        }
                      }
                    }
                  }
                }
              }
            }
          }
          frame "硬件版本读取" {
            n4223 = stacked-sequence {
              seq-local: [_ _ w5924 _] -> [_ _ _ w5931]
              frame #0 {
                w5920 = u8 137 ("命令")
                w5919 = u32 4 ("命令序号")
                n4224 = local read "设备索引号"() -> (w5922:u16)
                n4225 = local read "CAN卡类型"() -> (w5923:u32)
                n4226 = local read "CAN端口"() -> (w5921:u16)
                n4227 = local read "从板板号"() -> (w5917:u8)
                n4228 = local write "命令"(w5920) -> ()
                n4229 = call "多帧发送机制(EV05).vi"("can卡类型"=w5923, "设备索引号"=w5922, "CAN端口"=w5921, "命令"=w5920, "板号"=w5917, "命令序号"=w5919, "输入数据"=dbl[] [0.0]) -> ()  [unwired: 1 in, 12 out]
                n4230 = local write "命令序号"(w5919) -> ()
              }
              frame #1 {
              }
              frame #2 {
                n4231 = while {
                  tunnel: [w5925] -> w5924
                  i -> [w5930]
                  stop <- w5926 stop-if-true
                  n4232 = global read "EV05全局变量1.vi" "写入超时"() -> (w5925:bool)
                  n4233 = Greater Or Equal?(x=w5930, y=25) -> (x >= y?=w5927:bool)
                  n4234 = Or(x=w5925, y=w5927) -> (x .or. y?=w5926:bool)
                  n4235 = Wait Until Next ms Multiple(millisecond multiple=u32 100 ("毫秒倍数")) -> ()  [unwired: 1 out]
                }
              }
              frame #3 {
                n4236 = case shown="假" w5931 {
                  frame False {
                    n4237 = control-ref of="结果"() -> (w5933:refnum<vi>)
                    n4238 = Concatenate Strings("硬件版本" ("字符串"), "     读取失败" ("字符串")) -> (w5936:string)
                    n4239 = Build Array(w5936) -> (w5935:string[])
                    n4240 = call "表格编辑(版本读取).vi"("新元素/子数组"=w5935, "活动单元格:单元格背景色"=u32 16740749, "MCListbox引用句柄"=w5933) -> ()  [unwired: 9 out]
                  }
                  frame True {
                  }
                }
                n4241 = call <vilib>:"Unset Busy.vi"() -> ()  [unwired: 2 in, 10 out]
              }
            }
          }
          frame "写配置文件" {
            n4242 = disable-structure shown="启用" {
              frame Enabled {
                n4243 = local read "主从选择"() -> (w5945:enum32{"主板", "从板"})
                n4244 = case shown="\"主板\", 默认" w5945 {
                  tunnel: [w5964 w6155] -> w5948
                  tunnel: ["M0" w6161] -> w5946
                  frame "主板", Default {
                    n4245 = stacked-sequence {
                      seq-local: [w5978 _ _ _ _ _ _] -> [_ w6008 _ _ _ _ _]
                      seq-local: [string[] ["电池额定容量", "电池实际容量", "SOC", "SOH", "车牌号", "配置文件版本", "产品编号", "系统时钟"] _ _ _ _ _ _] -> [_ w6003 _ _ _ _ _]
                      seq-local: [_ _ _ _ string[] ["风机开启温度", "风机关闭温度", "加热开启温度", "加热关闭温度", "风机开启温差", "风机关闭温差", "加热关闭温差"] _ _] -> [_ _ _ _ _ w6107 _]
                      seq-local: [_ _ _ _ w6088 _ _] -> [_ _ _ _ _ w6105 _]
                      tunnel: [w5979 _ _ _ _ _ _] -> w5966
                      tunnel: [_ w6002 _ _ _ _ _] -> w5963
                      tunnel: [_ _ w6033 _ _ _ _] -> w5962
                      tunnel: [_ _ _ w6060 _ _ _] -> w5961
                      tunnel: [_ _ _ _ _ w6108 _] -> w5960
                      tunnel: [_ _ _ _ _ _ w6125] -> w5959
                      frame #0 {
                        w5970 = string[] ["", "", "", "", "", "", "", "", "", "", "  ", "", "", "", "", "", "", "", "", "", "  "]
                        n4246 = control-ref of="项目信息"() -> (w5998:refnum<vi>)
                        n4247 = property class="Tbl (严格)"(reference=w5998) -> ("Value"=w5974:string[][])  [unwired: 1 in, 2 out]
                        n4248 = control-ref of="项目信息2"() -> (w5992:refnum<vi>)
                        n4249 = Index Array(array=w5974, index (col)=0 ("禁用的索引 (列)")) -> (element=w5975:string[])  [unwired: 1 in]
                        n4250 = property class="Clust (严格)"(reference=w5992) -> ("Value"=w5991:T9)  [unwired: 1 in, 2 out]
                        n4251 = Index Array(array=w5974, index (col)=1 ("禁用的索引 (列)")) -> (element=w5973:string[])  [unwired: 1 in]
                        n4252 = local read "从板个数"() -> (w5997:dbl)
                        n4253 = Number To Decimal String(number=w5997) -> (decimal integer string=w5996:string)  [unwired: 1 out]
                        n4254 = Insert Into Array(array=w5975, new element=w5970) -> (w5972:string[])  [unwired: 1 in]
                        n4255 = Insert Into Array(array=w5973, new element=w5970) -> (w5971:string[])  [unwired: 1 in]
                        n4256 = Unbundle(w5991) -> ("电池额定容量(A)"=w5990:dbl, "电池实际容量(A)"=w5989:dbl, "车架(牌)号"=w5987:string, "配置文件版本"=w5986:string, "SOH(%)"=w5981:dbl, "SOC(%)"=w5980:dbl, "产品编号"=w5985:string, "系统时钟"=w5984:string)  [unwired: 1 out]
                        n4257 = Build Array("从板个数" ("元素"), w5996) -> (w5993:string[])
                        n4258 = Build Array(w5972, w5971) -> (w5968:string[][])
                        n4259 = Transpose 2D Array(2D array=w5968) -> (transposed array=w5967:string[][])
                        n4260 = Build Array(w5990, w5989, w5980, w5981) -> (w5988:dbl[])
                        n4261 = Build Array(w5987, w5986, w5985, w5984) -> (w5982:string[])
                        n4262 = for {
                          tunnel: w5988 -> [w6000] mode=indexing
                          tunnel: [w5999] -> w5983 mode=indexing
                          n4263 = Format Into String(format string="%#f" ("格式字符串"), w6000) -> (resulting string=w5999:string)  [unwired: 2 in, 1 out]
                        }
                        n4264 = Insert Into Array(array=w5967, index (row)=0 ("索引 (行)"), new element=w5993) -> (w5979:string[][])  [unwired: 1 in]
                        n4265 = Insert Into Array(array=w5983, new element=w5982) -> (w5978:string[])  [unwired: 1 in]
                      }
                      frame #1 {
                        n4266 = control-ref of="一级故障"() -> (w6029:refnum<vi>)
                        n4267 = property class="Clust (严格)"(reference=w6029) -> ("Value"=w6028:T10)  [unwired: 1 in, 2 out]
                        n4268 = Unbundle(w6028) -> ("总电压过高"=w6027:dbl, "整组电压不均衡"=w6022:dbl, "SOC过高"=w6015:dbl, "单体电压过高"=w6018:dbl, "总电压过低"=w6026:dbl, "温度过高"=w6025:dbl, "温度过低"=w6024:dbl, "单组电压不均衡"=w6023:dbl, "整组温度不均衡"=w6020:dbl, "单组温度不均衡"=w6021:dbl, "单体电压过低"=w6019:dbl, "充电电流过高"=w6017:dbl, "放电电流过高"=w6016:dbl, "SOC过低"=w6014:dbl, "内阻过大"=w6013:dbl, "极柱温度过高"=w6012:dbl, "SOH过低"=w6011:dbl)
                        n4269 = Build Array(w6027, w6026, w6025, w6024, w6023, w6022, w6021, w6020, w6018, w6019, w6017, w6016, w6015, w6014, w6013, w6012, w6011) -> (w6010:dbl[])
                        n4270 = for {
                          tunnel: w6010 -> [w6031] mode=indexing
                          tunnel: [w6030] -> w6007 mode=indexing
                          n4271 = Format Into String(format string="%#f" ("格式字符串"), w6031) -> (resulting string=w6030:string)  [unwired: 2 in, 1 out]
                        }
                        n4272 = Insert Into Array(array=w6008, new element=w6007) -> (w6006:string[])  [unwired: 1 in]
                        n4273 = Insert Into Array(array=w6003, new element=string[] ["总电压过高一级", "总电压过低一级", "温度过高一级", "温度过低一级", "单组电压不均衡一级", "整组电压不均衡一级", "单组温度不均衡一级", "整组温度不均衡一级", "单体电压过高一级", "单体电压过低一级", "充电电流过高一级", "放电电流过高一级", "SOC过高一级", "SOC过低一级", "内阻过大一级", "极柱温度过高一级", "SOH过低一级"]) -> (w6005:string[])  [unwired: 1 in]
                        n4274 = Build Array(w6005, w6006) -> (w6004:string[][])
                        n4275 = Transpose 2D Array(2D array=w6004) -> (transposed array=w6002:string[][])
                      }
                      frame #2 {
                        n4276 = control-ref of="一级故障 2"() -> (w6034:refnum<vi>)
                        n4277 = property class="Clust (严格)"(reference=w6034) -> ("Value"=w6056:T10)  [unwired: 1 in, 2 out]
                        n4278 = Unbundle(w6056) -> ("总电压过高"=w6055:dbl, "整组电压不均衡"=w6050:dbl, "SOC过高"=w6043:dbl, "单体电压过高"=w6046:dbl, "总电压过低"=w6054:dbl, "温度过高"=w6053:dbl, "温度过低"=w6052:dbl, "单组电压不均衡"=w6051:dbl, "整组温度不均衡"=w6048:dbl, "单组温度不均衡"=w6049:dbl, "单体电压过低"=w6047:dbl, "充电电流过高"=w6045:dbl, "放电电流过高"=w6044:dbl, "SOC过低"=w6042:dbl, "内阻过大"=w6041:dbl, "极柱温度过高"=w6040:dbl, "SOH过低"=w6039:dbl)
                        n4279 = Build Array(w6055, w6054, w6053, w6052, w6051, w6050, w6049, w6048, w6046, w6047, w6045, w6044, w6043, w6042, w6041, w6040, w6039) -> (w6038:dbl[])
                        n4280 = for {
                          tunnel: w6038 -> [w6058] mode=indexing
                          tunnel: [w6057] -> w6037 mode=indexing
                          n4281 = Format Into String(format string="%#f" ("格式字符串"), w6058) -> (resulting string=w6057:string)  [unwired: 2 in, 1 out]
                        }
                        n4282 = Build Array(string[] ["总电压过高二级", "总电压过低二级", "温度过高二级", "温度过低二级", "单组电压不均衡二级", "整组电压不均衡二级", "单组温度不均衡二级", "整组温度不均衡二级", "单体电压过高二级", "单体电压过低二级", "充电电流过高二级", "放电电流过高二级", "SOC过高二级", "SOC过低二级", "内阻过大二级", "极柱温度过高二级", "SOH过低二级"], w6037) -> (w6035:string[][])
                        n4283 = Transpose 2D Array(2D array=w6035) -> (transposed array=w6033:string[][])
                      }
                      frame #3 {
                        n4284 = control-ref of="一级故障 3"() -> (w6061:refnum<vi>)
                        n4285 = property class="Clust (严格)"(reference=w6061) -> ("Value"=w6083:T10)  [unwired: 1 in, 2 out]
                        n4286 = Unbundle(w6083) -> ("总电压过高"=w6082:dbl, "整组电压不均衡"=w6077:dbl, "SOC过高"=w6070:dbl, "单体电压过高"=w6073:dbl, "总电压过低"=w6081:dbl, "温度过高"=w6080:dbl, "温度过低"=w6079:dbl, "单组电压不均衡"=w6078:dbl, "整组温度不均衡"=w6075:dbl, "单组温度不均衡"=w6076:dbl, "单体电压过低"=w6074:dbl, "充电电流过高"=w6072:dbl, "放电电流过高"=w6071:dbl, "SOC过低"=w6069:dbl, "内阻过大"=w6068:dbl, "极柱温度过高"=w6067:dbl, "SOH过低"=w6066:dbl)
                        n4287 = Build Array(w6082, w6081, w6080, w6079, w6078, w6077, w6076, w6075, w6073, w6074, w6072, w6071, w6070, w6069, w6068, w6067, w6066) -> (w6065:dbl[])
                        n4288 = for {
                          tunnel: w6065 -> [w6085] mode=indexing
                          tunnel: [w6084] -> w6064 mode=indexing
                          n4289 = Format Into String(format string="%#f" ("格式字符串"), w6085) -> (resulting string=w6084:string)  [unwired: 2 in, 1 out]
                        }
                        n4290 = Build Array(string[] ["总电压过高三级", "总电压过低三级", "温度过高三级", "温度过低三级", "单组电压不均衡三级", "整组电压不均衡三级", "单组温度不均衡三级", "整组温度不均衡三级", "单体电压过高三级", "单体电压过低三级", "充电电流过高三级", "放电电流过高三级", "SOC过高三级", "SOC过低三级", "内阻过大三级", "极柱温度过高三级", "SOH过低三级"], w6064) -> (w6062:string[][])
                        n4291 = Transpose 2D Array(2D array=w6062) -> (transposed array=w6060:string[][])
                      }
                      frame #4 {
                        n4292 = control-ref of="加热控制参数"() -> (w6098:refnum<vi>)
                        n4293 = property class="Clust (严格)"(reference=w6098) -> ("Value"=w6097:T11)  [unwired: 1 in, 2 out]
                        n4294 = Unbundle(w6097) -> ("风机开启温度"=w6096:dbl, "风机关闭温度"=w6095:dbl, "加热开启温度"=w6094:dbl, "加热关闭温度"=w6093:dbl, "风机开启温差"=w6092:dbl, "风机关闭温差"=w6091:dbl, "加热关闭温差"=w6087:dbl)
                        n4295 = Build Array(w6096, w6095, w6094, w6093, w6092, w6091, w6087) -> (w6090:dbl[])
                        n4296 = for {
                          tunnel: w6090 -> [w6100] mode=indexing
                          tunnel: [w6099] -> w6088 mode=indexing
                          n4297 = Format Into String(format string="%#f" ("格式字符串"), w6100) -> (resulting string=w6099:string)  [unwired: 2 in, 1 out]
                        }
                      }
                      frame #5 {
                        n4298 = control-ref of="充电控制参数"() -> (w6118:refnum<vi>)
                        n4299 = property class="Clust (严格)"(reference=w6118) -> ("Value"=w6120:T12)  [unwired: 1 in, 2 out]
                        n4300 = Unbundle(w6120) -> ("最大允许单体电压"=w6117:dbl, "最大允许总电压"=w6116:dbl, "最小允许单体电压"=w6115:dbl, "最大允许充电电流"=w6114:dbl, "最小允许充电电流"=w6113:dbl, "最大允许充电温度"=w6112:dbl, "最小允许充电温度"=w6111:dbl, "电流步长"=w6110:dbl)
                        n4301 = Build Array(w6117, w6116, w6115, w6114, w6113, w6112, w6111, w6110) -> (w6119:dbl[])
                        n4302 = for {
                          tunnel: w6119 -> [w6122] mode=indexing
                          tunnel: [w6121] -> w6104 mode=indexing
                          n4303 = Format Into String(format string="%#f" ("格式字符串"), w6122) -> (resulting string=w6121:string)  [unwired: 2 in, 1 out]
                        }
                        n4304 = Insert Into Array(array=w6105, new element=w6104) -> (w6103:string[])  [unwired: 1 in]
                        n4305 = Insert Into Array(array=w6107, new element=string[] ["最大允许单体电压", "最大允许总电压", "最小允许单体电压", "最大允许充电电流", "最小允许充电电流", "最大允许充电温度", "最小允许充电温度", "电流步长"]) -> (w6102:string[])  [unwired: 1 in]
                        n4306 = Build Array(w6102, w6103) -> (w6109:string[][])
                        n4307 = Transpose 2D Array(2D array=w6109) -> (transposed array=w6108:string[][])
                      }
                      frame #6 {
                        n4308 = control-ref of="电池信息"() -> (w6146:refnum<vi>)
                        n4309 = property class="Clust (严格)"(reference=w6146) -> ("Value"=w6149:T13)  [unwired: 1 in, 2 out]
                        n4310 = Unbundle(w6149) -> ("电池串联"=w6145:dbl, "电池并联"=w6144:dbl, "累计放电总安时"=w6142:dbl, "电池包额定容量"=w6141:dbl, "电池包额定能量(kWh)"=w6140:dbl, "电池包额定总电压"=w6139:dbl, "累计充电总安时"=w6143:dbl, "电池充满次数"=w6138:dbl, "电池放空次数"=w6137:dbl, "电池充电次数"=w6136:dbl, "电池生产日期"=w6134:string, "电池厂家"=w6133:string, "电池类型"=w6132:string, "电池包组号"=w6131:string, "电池包产权标识"=w6130:string, "电池应用车型"=w6129:string, "实际容量"=w6124:dbl)
                        n4311 = Build Array(w6134, w6133, w6132, w6131, w6130, w6129) -> (w6128:string[])
                        n4312 = Build Array(w6145, w6144, w6143, w6142, w6141, w6140, w6139, w6138, w6137, w6136, w6124) -> (w6135:dbl[])
                        n4313 = for {
                          tunnel: w6135 -> [w6151] mode=indexing
                          tunnel: [w6150] -> w6127 mode=indexing
                          n4314 = Format Into String(format string="%#f" ("格式字符串"), w6151) -> (resulting string=w6150:string)  [unwired: 2 in, 1 out]
                        }
                        n4315 = Insert Into Array(array=w6128, new element=w6127) -> (w6126:string[])  [unwired: 1 in]
                        n4316 = call <vilib>:"Unset Busy.vi"() -> ()  [unwired: 2 in, 10 out]
